vi "Read Power.vi"(0 "SG Path Power Meter Accessor in":refnum<class "SG Path Simulated PM Accessor.lvclass">, 5 "Cal point in":T1, 11 "error in":errorcluster) -> (4 "SG Path Power Meter Accessor out":refnum<class "SG Path Simulated PM Accessor.lvclass">, 6 "Power (dBm)":dbl, 15 "error out":errorcluster)   [LabVIEW 2023, in "RFFixtureCharact.Instruments.lvlib" / "SG Path Simulated PM Accessor.lvclass"]
uses:
  SG Path Simulated PM Accessor.lvclass
  Public/Base Classes/Scalar/Scalar Path/Type Definitions/Cal Point.ctl
  Public/Base Classes/Scalar/Scalar Path/Scalar Path.lvclass
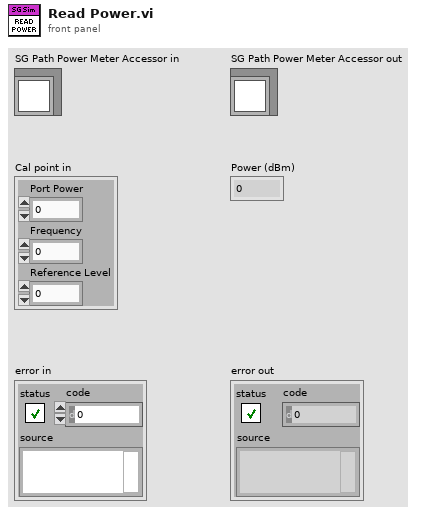
[diagram p1: front panel]
types:
  T1 = typedef "RFFixtureCharact.Public.lvlib/Scalar Path.lvclass/Cal Point.ctl" = cluster{"Port Power":dbl, "Frequency":dbl, "Reference Level":dbl}
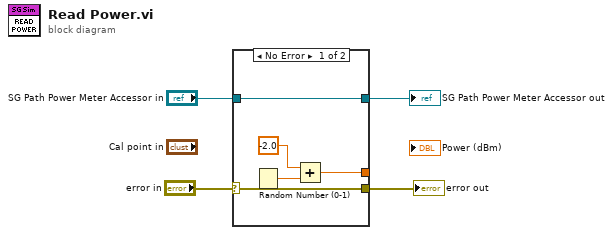
[diagram p0: block diagram]
diagram:
  n1 = case shown="No Error" "error in" {
    selector: "error in" -> [w9 w11]
    tunnel: [w9 w11] -> w1
    tunnel: [w5 _] -> _
    tunnel: [w8 w10] -> w3
    tunnel: "SG Path Power Meter Accessor in" -> [w8 w10]
    frame No Error {
      n2 = Random Number (0-1)() -> (number: 0 to 1=w6:dbl)
      n3 = Add(x=-2.0 ("power"), y=w6) -> (x+y=w5:dbl)
    }
    frame Error {
    }
  }
  "error out" <- w1
  "SG Path Power Meter Accessor out" <- w3
